vi "Logging.vi"(0 "Logger in":refnum<class "Generic Logger.lvclass">, 5 "Log Level":T1, 7 "Caller":string, 9 "Content":string, 11 "error in (no error)":errorcluster) -> (4 "Logger out":refnum<class "Generic Logger.lvclass">, 15 "error out":errorcluster)   [LabVIEW 2020, in "Logging.lvlib" / "Generic Logger.lvclass"]
uses:
  Generic Logger.lvclass
  Define/Log Level.ctl
  Generic Logger.lvclass/Generic Logger.ctl
  Logging.lvlib
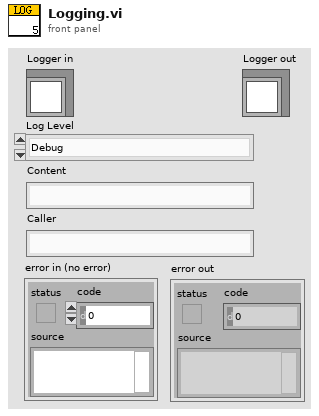
[diagram p1: front panel]
types:
  T1 = typedef "Logging.lvlib/Log Level.ctl" = enum16{"Debug", "Info", "Warn", "Error"}
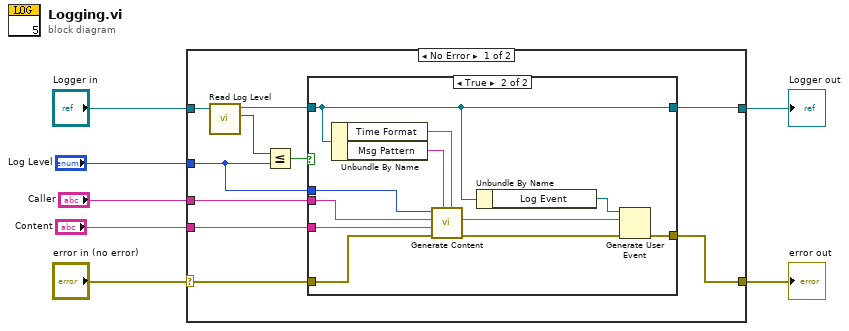
[diagram p0: block diagram]
diagram:
  n1 = case shown="No Error" "error in (no error)" {
    selector: "error in (no error)" -> [w17 w32]
    tunnel: [w16 w32] -> w6
    tunnel: [w13 w31] -> w4
    tunnel: "Logger in" -> [w15 w31]
    tunnel: "Content" -> [w10 _]
    tunnel: "Log Level" -> [w9 _]
    tunnel: "Caller" -> [w8 _]
    frame No Error {
      n2 = call-dynamic "Read Log Level.vi"("Logger in"=w15) -> ("Log Level"=w11:T1, "Logger out"=w14:refnum<class "Generic Logger.lvclass">)  [unwired: 8 in, 1 out]
      n3 = Less Or Equal?(x=w11, y=w9) -> (x <= y?=w12:bool)
      n4 = case shown="True" w12 {
        tunnel: w10 -> [_ w26]
        tunnel: w17 -> [w19 w25]
        tunnel: [w19 w29] -> w16
        tunnel: w14 -> [w18 w22]
        tunnel: [w18 w22] -> w13
        tunnel: w9 -> [_ w28]
        tunnel: w8 -> [_ w27]
        frame False {
        }
        frame True {
          n5 = Unbundle By Name(w22) -> ("Time Format"=w20:string, "Msg Pattern"=w21:string)
          n6 = call "Generate Content.vi"("Time Format"=w20, "Msg Pattern"=w21, "error in (no error)"=w25, "Msg"=w26, "Caller"=w27, "Log Level"=w28) -> ("error out"=w24:errorcluster, "Content"=w23:string)  [unwired: 4 in]
          n7 = Unbundle By Name(w22) -> ("Log Event"=w30:refnum<user-event>)
          n8 = Generate User Event(user event=w30, event data cluster=w23, error in=w24) -> (error out=w29:errorcluster)  [unwired: 1 in, 1 out]
        }
      }
    }
    frame Error {
    }
  }
  "error out" <- w6
  "Logger out" <- w4
